vi "WholeImageROIFitBackUp.vi"(3 "Select directory with EYE files":path=path "E:/junk/EYEFiles") -> ()   [LabVIEW 2022 SP3]
uses:
  <vilib>/Utility/file.llb/Read From Spreadsheet File (DBL).vi
  <vilib>/Utility/file.llb/Write To Spreadsheet File (DBL).vi
  <vilib>/Analysis/NI_AALBase.lvlib
  <vilib>/Analysis/baseanly.llb/Mean (DBL).vi
panel:
  out "Sector as data array":dbl[][](graph)
  out "min value":dbl
  out "max value":dbl
  in  "ExitSendCmd":bool
  in  "Calculate TTIs":bool
  out "Current File":string
  out "Col scores":dbl[][](graph)
  out "Col midband":dbl[][](graph)
  out "NN Score":dbl[][](graph)
  in  "Tab Control":T1(tab)=enum."Image Prams"
  in  "Corrections":T2(ring)=enum."att correction"
  in  "type of cal file":u16(ring) items=["Normal Cal File", "Cross Cal File", "No cal file"]
  out "Cal File Att":string
  out "RF File Att":string
  in  "Cal File Name":string
  in  "Fit band":T3 {"center freq" format="%.2f"; "stop freq" format="%.2f"; "start" format="%.2f"}
  in  "Use Info In Header?":bool=TRUE
  in  "Lines to Avg":i32=1
  in  "Pts between window":i32=8
  in  "Pts in window":i32=64
  in  "sound speed":dbl=1.5 format="%.2f"
  in  "Padded FFT size":u16(ring)=6 items=["next 2^n", "8", "16", "32", "64", "128", "256", "512"]
  in  "Att (db/ cm MHz)":dbl=0.5 format="%.2f"
  in  "Add Switch Noise?":bool
  in  "Log scaling?":bool=TRUE
  out "Fit array":T4
  in  "Sub-Band Filter":T5={"Fit band"={"low freq"=3.5, "high freq"=8.0, "center freq"=5.75}, "MB threshold"=0.0, "Sub-Band Filter?"=FALSE} {"MB threshold" format="%.2f"; "Fit band"."center freq" format="%.2f"; "Fit band"."high freq" format="%.2f"; "Fit band"."low freq" format="%.2f"}
  in  "CQPrams":T6={"Data System params"={"sample freq (MHz)"=50.0, "focal length (mm)"=32.0, "aperature radius (mm)"=3.5, "pts in window"=64.0}, "Show CQ^2 image?"=FALSE, "Save?"=FALSE} {"Data System params"."pts in window" format="%.2f"; "Data System params"."aperature radius (mm)" format="%.2f"; "Data System params"."focal length (mm)" format="%.2f"; "Data System params"."sample freq (MHz)" format="%.2f"}
  out "CQ^2":ext[][](graph)
  out "radius (micron)":sgl[][](graph)
  in  "Range Params":T7={"mb max"=-20.0, "mb min"=-70.0, "slope max"=8.0, "slope min"=-8.0, "int max"=5.0, "int min"=-85.0} {"int min" format="%.2f"; "int max" format="%.2f"; "slope min" format="%.2f"; "slope max" format="%.2f"; "mb min" format="%.2f"; "mb max" format="%.2f"}
  in  "Final Sector Image Size":T8={"x"=346, "y"=240, "Trim image sides?"=FALSE, "start trim"=45, "end trim line"=256}
  in  "Simple BMP":bool
  in  "Raw Data Formats":T9(ring)
  in  "Save Raw Results?":bool
  in  "PSA Value":dbl=8.7 format="%.2f"
  in  "Look Up Table":path=path "E:/junk/EYEFiles/99lktbl10-31.txt"
  in  "Create Score Image?":bool
  in  "thresholds":T10={"T1"=0.37, "T2"=0.38, "T3"=0.39, "T4"=0.4, "T5"=0.43} {"T5" scale=3.0..47.0; "T4" scale=3.0..47.0; "T3" scale=3.0..47.0; "T2" scale=3.0..47.0; "T1" scale=3.0..47.0}
  in  "Save Score Dat?":bool
  in  "Color Table":u32[](array[colorbox])=[0, 0, 65793, 131586, 197379, 263172, 328965, 394758, 460551, 526344, 592137, 657930, 723723, 789516, 855309, 921102, 986895, 1052688, 1118481, 1184274, 1250067, 1315860, 1381653, 1447446, 1513239, 1579032, 1644825, 1710618, 1776411, 1842204, 1907997, 1973790, 2039583, 2105376, 2171169, 2236962, 2302755, 2368548, 2434341, 2500134, 2565927, 2631720, 2697513, 2763306, 2829099, 2894892, 2960685, 3026478, 3092271, 3158064, 3223857, 3289650, 3355443, 3421236, 3487029, 3552822, 3618615, 3684408, 3750201, 3815994, 3881787, 3947580, 4013373, 4079166, 4144959, 4210752, 4276545, 4342338, 4408131, 4473924, 4539717, 4605510, 4671303, 4737096, 4802889, 4868682, 4934475, 5000268, 5066061, 5131854, 5197647, 5263440, 5329233, 5395026, 5460819, 5526612, 5592405, 5658198, 5723991, 5789784, 5855577, 5921370, 5987163, 6052956, 6118749, 6184542, 6250335, 6316128, 6381921, 6447714, 6513507, 6579300, 6645093, 6710886, 6776679, 6842472, 6908265, 6974058, 7039851, 7105644, 7171437, 7237230, 7303023, 7368816, 7434609, 7500402, 7566195, 7631988, 7697781, 7763574, 7829367, 7895160, 7960953, 8026746, 8092539, 8158332, 8224125, 8289918, 8355711, 8421504, 8487297, 8553090, 8618883, 8684676, 8750469, 8816262, 8882055, 8947848, 9013641, 9079434, 9145227, 9211020, 9276813, 9342606, 9408399, 9474192, 9539985, 9605778, 9671571, 9737364, 9803157, 9868950, 9934743, 10000536, 10066329, 10132122, 10197915, 10263708, 10329501, 10395294, 10461087, 10526880, 10592673, 10658466, 10724259, 10790052, 10855845, 10921638, 10987431, 11053224, 11119017, 11184810, 11250603, 11316396, 11382189, 11447982, 11513775, 11579568, 11645361, 11711154, 11776947, 11842740, 11908533, 11974326, 12040119, 12105912, 12171705, 12237498, 12303291, 12369084, 12434877, 12500670, 12566463, 12632256, 12698049, 12763842, 12829635, 12895428, 12961221, 13027014, 13092807, 13158600, 13224393, 13290186, 13355979, 13421772, 13487565, 13553358, 13619151, 13684944, 13750737, 13816530, 13882323, 13948116, 14013909, 14079702, 14145495, 14211288, 14277081, 14342874, 14408667, 14474460, 14540253, 14606046, 14671839, 14737632, 14803425, 14869218, 14935011, 15000804, 15066597, 15132390, 15198183, 15263976, 15329769, 15395562, 15461355, 15527148, 15592941, 15658734, 15724527, 15790320, 15856113, 15921906, 15987699, 16053492, 16119285, 16185078, 16250871, 16316664, 16382457, 6352640, 12058434, 16770066, 16758546, 16711731]
  in  "Data Set":i32
  in  "Rescale Thresh":bool
  in  "Create Cross Cal?":bool
  out "Cross Cal":dbl[][](graph)
  in  "Ring":u16(ring) items=["Select Files in Listbox", "Choose list of files"]
  in  "File Names":i32[](listbox)
  out "raw data":i16[][](graph)
  out "midband fit":dbl[][](graph)
  out "intercept":dbl[][](graph)
  out "slope":dbl[][](graph)
  # "© 2000-2010 Riverside Research Institute"
  # "Parameters to select before hitting \"Calculate TTIs\"."
  # "Spectrum Fit Parameters"
  # "Select to add back in switch noise from B&K Hawk machine."
  # "Values used to make image."
  # "Optional suband filter which is really never used and may not function properly in current version."
  # "Can be selected after calculating TTIs"
  # "CQPrams files are saved as spreadsheet files. Radius file is in microns and cq^2 file is in dB."
  # "Save raw data and MB side by side"
  # "Score images need to be created with all corrections applied data. This means a cross cal file with attenutation corrections for Hawk and Hitachi, and data base corrections for B&K 3535.\n\nFinal image size settings are in Image Prams tab. Data saves as a BMP file in sector format.\n\nCreate Score Image? will color code images and Save Score Dat? will save images as BMPs."
  # "If making Cross Cal file, select No cal file option and att correction."
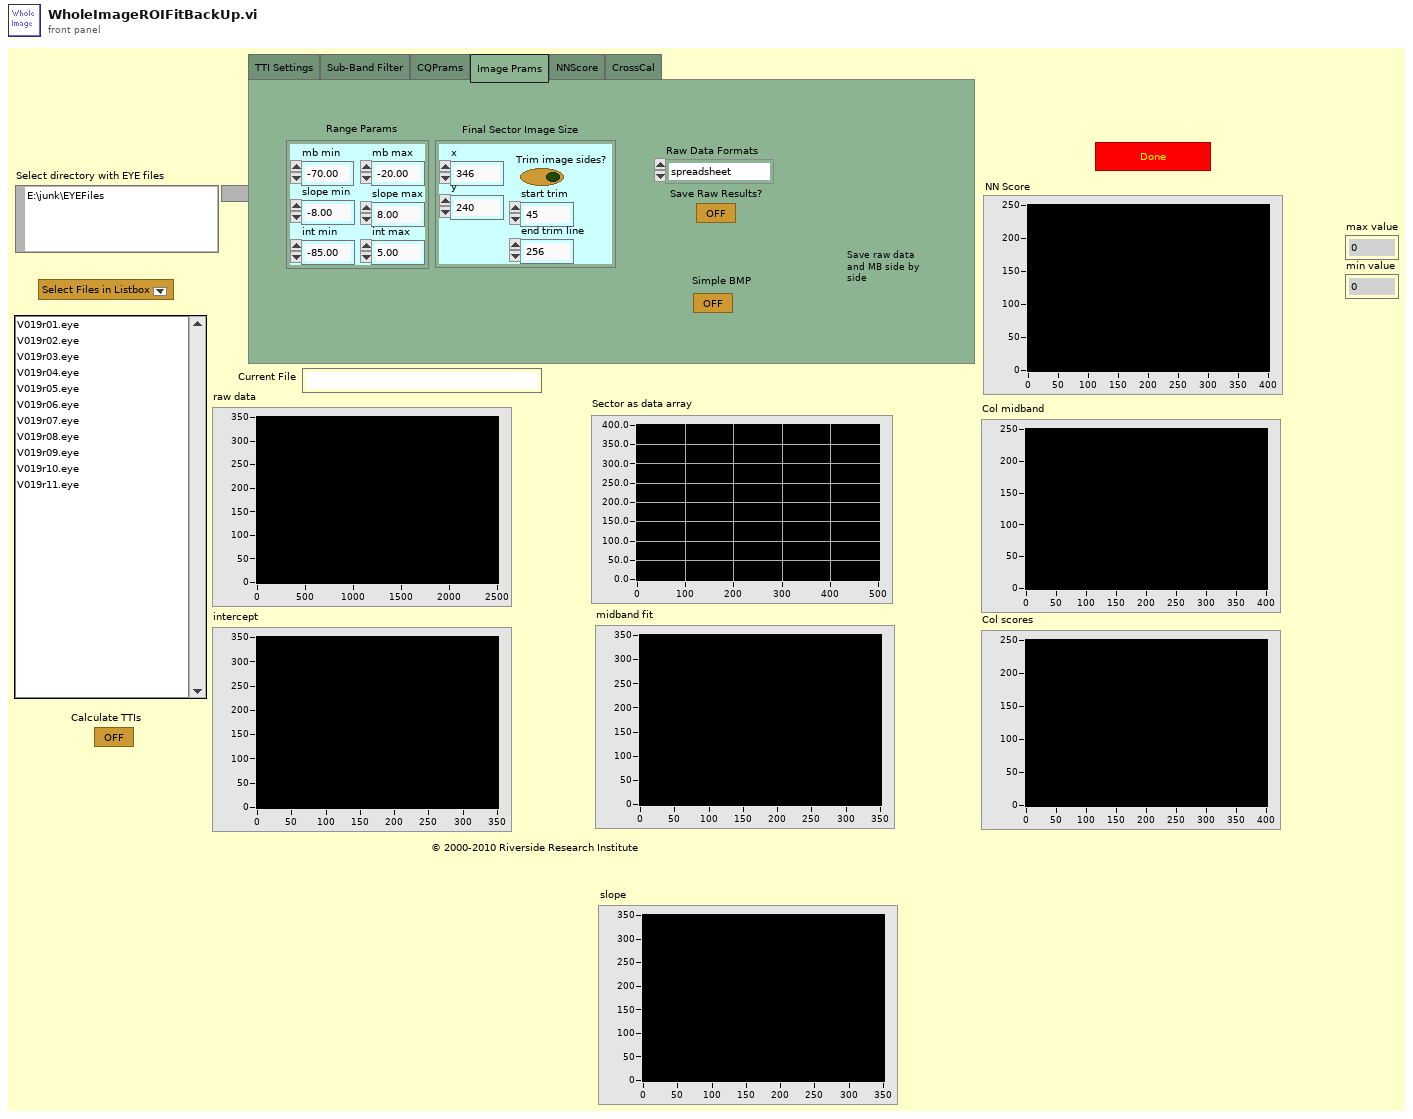
[diagram p1: front panel]
types:
  T1 = enum32{"TTI Settings", "Sub-Band Filter", "CQPrams", "Image Prams", "NNScore", "CrossCal"}
  T2 = enum16{"no att correction", "att correction", "B&K 3535, TGC & att corr"}
  T3 = cluster{"start":dbl, "stop freq":dbl, "center freq":dbl}
  T4 = cluster{"x length":i32, "y length":i32, "ROIs in x":i32, "ROIs in y":i32}
  T5 = cluster{"Fit band":cluster{"low freq":dbl, "high freq":dbl, "center freq":dbl}, "MB threshold":dbl, "Sub-Band Filter?":bool}
  T6 = cluster{"Data System params":cluster{"sample freq (MHz)":dbl, "focal length (mm)":sgl, "aperature radius (mm)":sgl, "pts in window":dbl}, "Show CQ^2 image?":bool, "Save?":bool}
  T7 = cluster{"mb max":dbl, "mb min":dbl, "slope max":dbl, "slope min":dbl, "int max":dbl, "int min":dbl}
  T8 = cluster{"x":i32, "y":i32, "Trim image sides?":bool, "start trim":i32, "end trim line":i32}
  T9 = enum16{"spreadsheet", "8 bit byte file", "sector byte file", "8 bit BMP file", "sector 8 bit BMP file"}
  T10 = cluster{"T1":dbl, "T2":dbl, "T3":dbl, "T4":dbl, "T5":dbl}
  T11 = cluster{"# rf points per line":u16, "# lines per scan":u16, "sample rate MHz":u16, "# A/D bits":u16, "# bytes per A/D":u16, "TGC Flag":u16, "A/D Type":string}
  T12 = cluster{"bandwidth":sgl, "center freq":sgl, "start freq":sgl, "ID":i32}
  T13 = cluster{"delay":sgl, "pivot distance":sgl, "sector scan angle":sgl, "operator":string, "Scan Mode":string, "location":string}
  T14 = cluster{"RF file name":string, "RF file att":string, "RF cal file name":string, "RF cal file att":string}
  T15 = cluster{"RF cal file name":string, "RF file att":string, "Cal File Name":string, "RF cal file att":string}
  T16 = cluster{"start freq":sgl, sgl, "center freq":sgl}
  T17 = cluster{"Pts in window":i32, "Lines to Avg":i32, dbl, "# lines per scan":u16}
  T18 = cluster{"slope (m)":dbl[][], "intercept (b)":dbl[][], "midband fit":dbl[][], "pts in fit":dbl}
  T19 = cluster{"slope (m)":dbl, "m stand dev":dbl, "intercept (b)":dbl, "b stand dev":dbl, "MSE":dbl, "midband fit":dbl, "pts in fit":dbl}
  T20 = typedef "imagedata.ctl" = cluster{"image type":i32, "image depth":i32, "image":u8[], "mask":u8[], "colors":u32[], "Rectangle":cluster{"left":i16, "top":i16, "right":i16, "bottom":i16}}
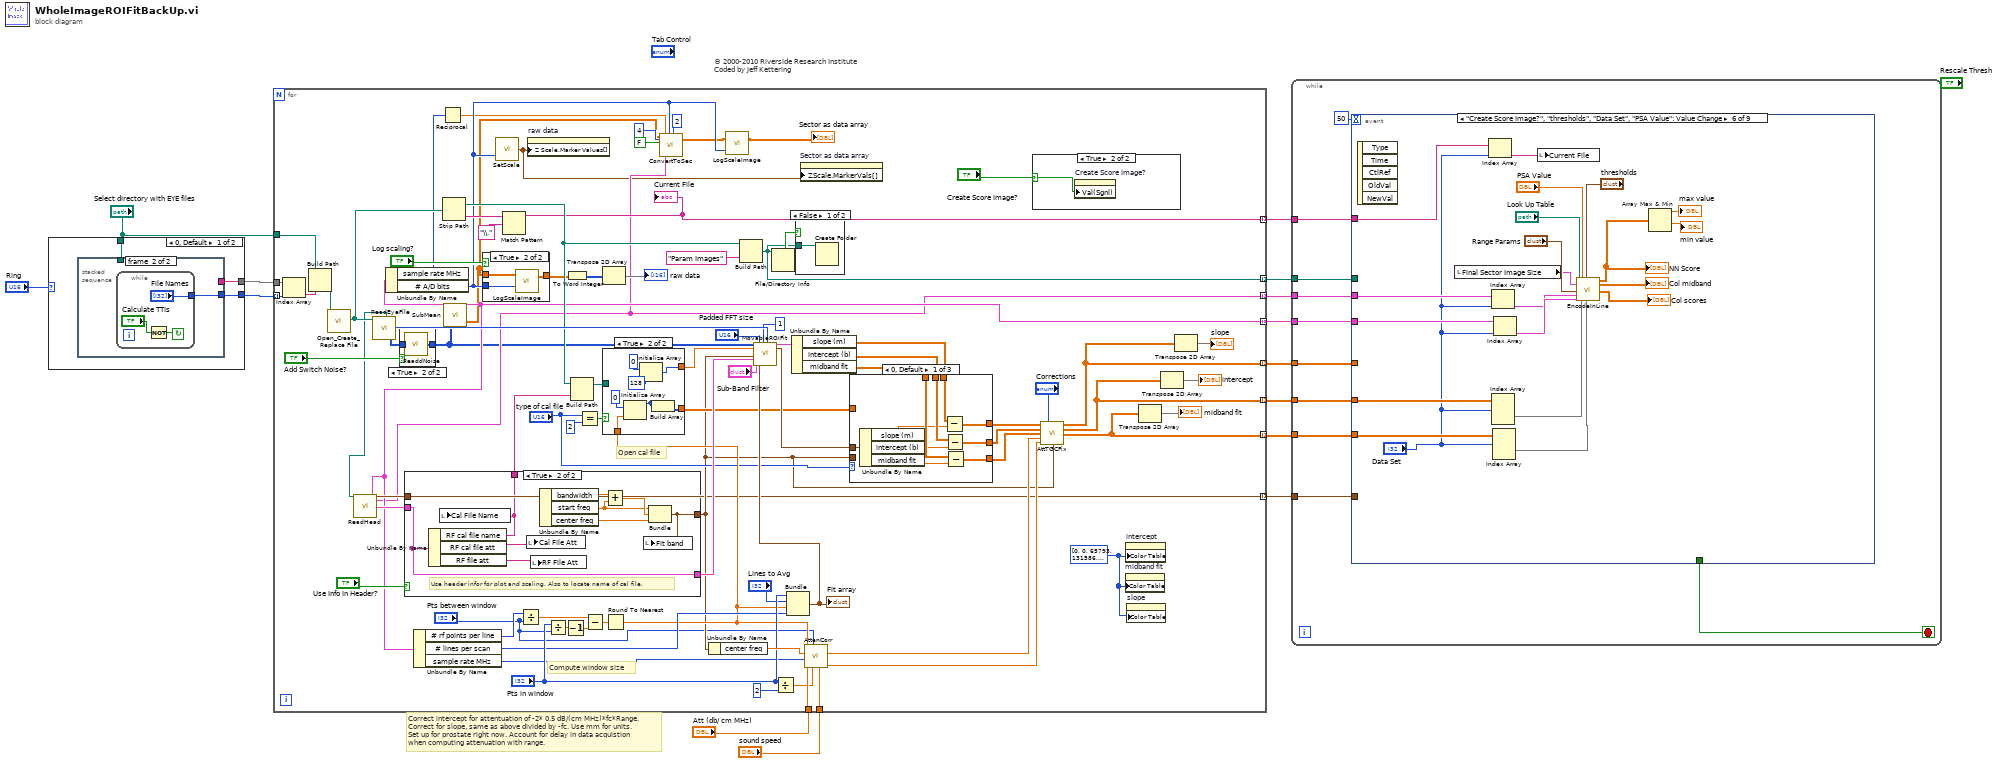
[diagram p0: block diagram]
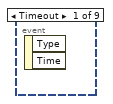
[diagram p2: hidden frame]
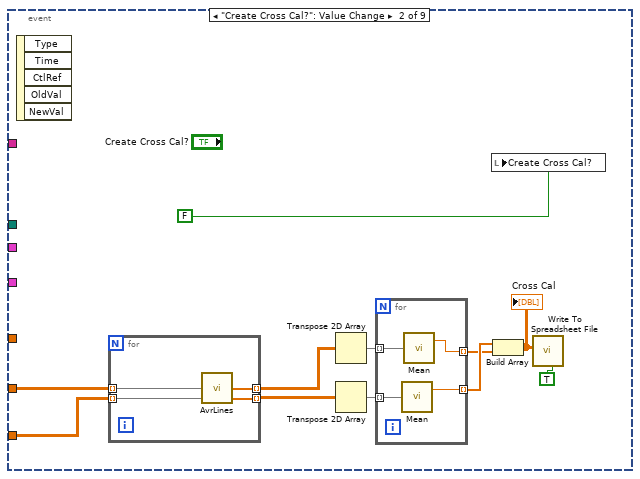
[diagram p3: hidden frame]
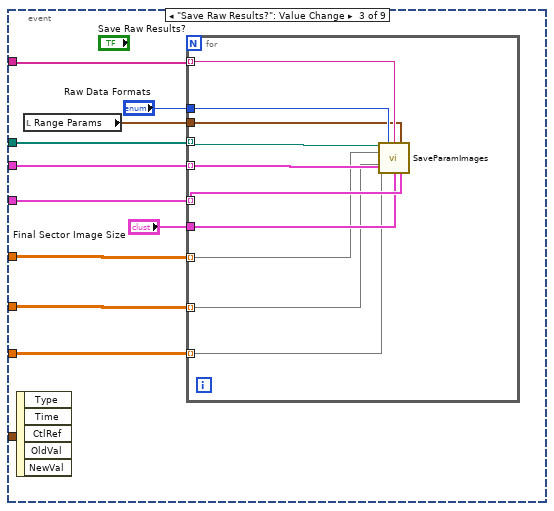
[diagram p4: hidden frame]
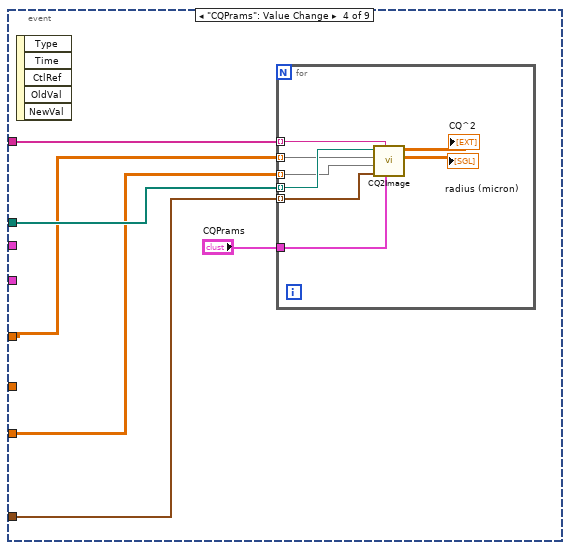
[diagram p5: hidden frame]
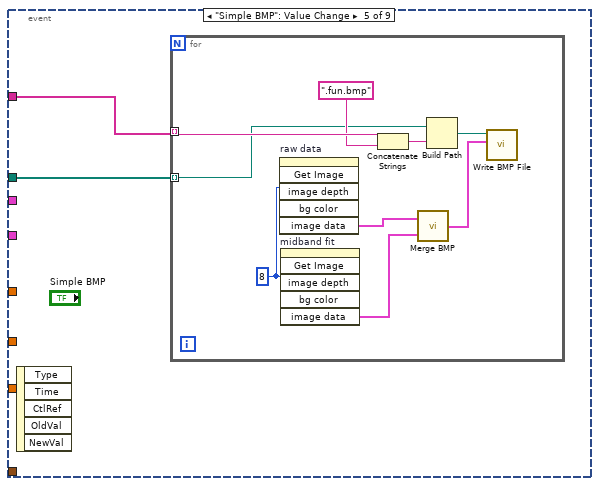
[diagram p6: hidden frame]
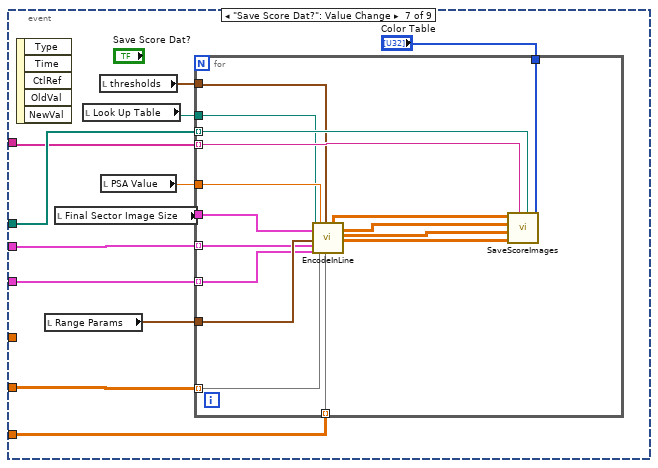
[diagram p7: hidden frame]
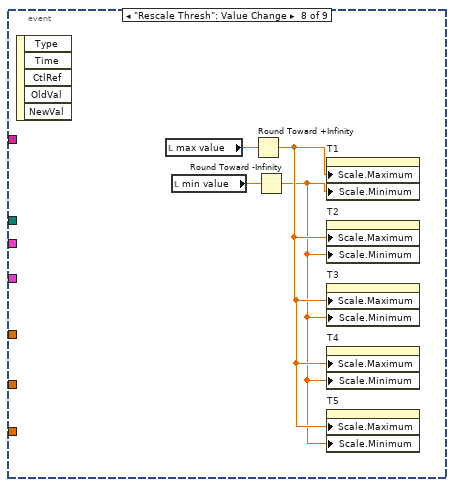
[diagram p8: hidden frame]
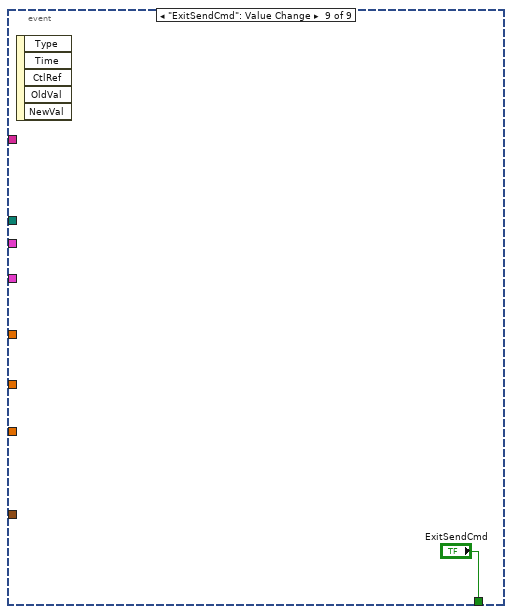
[diagram p9: hidden frame]
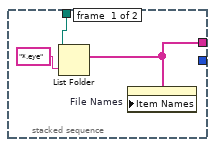
[diagram p10: hidden frame]
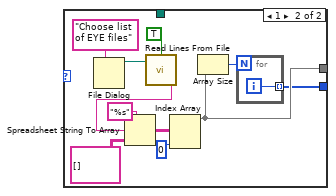
[diagram p11: hidden frame]
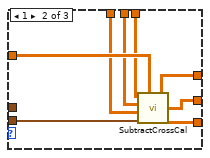
[diagram p15: hidden frame]
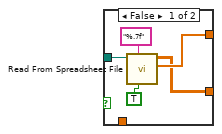
[diagram p17: hidden frame]
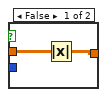
[diagram p18: hidden frame]
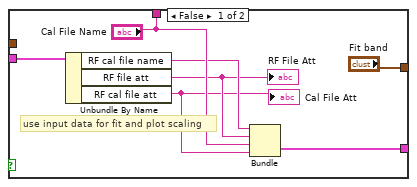
[diagram p19: hidden frame]
diagram:
  # "© 2000-2010 Riverside Research Institute\nCoded by Jeff Kettering"
  # "Correct intercept for attentuation of -2* 0.5 dB/(cm MHz)*fc*Range.\nCorrect for slope, same as above divided by -fc. Use mm for units. \nSet up for prostate right now. Account for delay in data acquistion when computing attenuation with range."
  n1 = case shown="0, Default" "Ring" {
    tunnel: [w17 w27] -> w14
    tunnel: "Select directory with EYE files" -> [w16 _]
    tunnel: [w15 w25] -> w13
    frame 0, Default {
      n2 = stacked-sequence {
        tunnel: [w19 _] -> w17
        tunnel: w16 -> [w18 _]
        tunnel: [_ w21] -> w15
        frame #0 {
          n3 = List Folder(path=w18, pattern="*.eye") -> (filenames=w19:string[])  [unwired: 1 in, 4 out]
          n4 = property on="File Names" class="LstBox (strict)"("Item Names"=w19) -> ()  [unwired: 2 in, 2 out]
        }
        frame #1 {
          n5 = while {
            tunnel: ["File Names"] -> w21
            stop <- w22 continue-if-true
            n6 = Not(x="Calculate TTIs") -> (.not. x?=w22:bool)
          }
        }
      }
    }
    frame 1 {
      n7 = File Dialog(7:"Choose list of EYE files" ("prompt")) -> (3:w33:path)  [unwired: 1 in, 8 out]
      n8 = call <vilib>:"Read Lines From File.vi"("convert eol? (no:F)"=TRUE, "file path (dialog if empty)"=w33) -> ("line string"=w28:string)  [unwired: 1 in, 6 out]
      n9 = Spreadsheet String To Array(format string="%s", spreadsheet string=w28, array type (2D Dbl)=string[][] [] ("Array Constant")) -> (array=w32:string[][])  [unwired: 1 in]
      n10 = Index Array(array=w32, index (col)=0) -> (element=w27:string[])  [unwired: 1 in]
      n11 = Array Size(array=w27) -> (size(s)=w26:i32)
      n12 = for {
        N: w26 -> [_]
        tunnel: [w36] -> w25 mode=indexing
        i -> [w36]
      }
    }
  }
  n13 = for {
    tunnel: w14 -> [w111]
    tunnel: "Select directory with EYE files" -> [w110]
    tunnel: w13 -> [w106] mode=indexing
    tunnel: "Att (db/ cm MHz)" -> [w96]
    tunnel: "sound speed" -> [w68]
    tunnel: [w61] -> w8 mode=indexing
    tunnel: [w60] -> w7 mode=indexing
    tunnel: [w55] -> w6 mode=indexing
    tunnel: [w56] -> w5 mode=indexing
    tunnel: [w57] -> w4 mode=indexing
    tunnel: [w54] -> w3 mode=indexing
    tunnel: [w46] -> w2 mode=indexing
    tunnel: [w53] -> w1 mode=indexing
    w67 = u32[] [0, 0, 65793, 131586, 197379, 263172, 328965, 394758, 460551, 526344, 592137, 657930, 723723, 789516, 855309, 921102, 986895, 1052688, 1118481, 1184274, 1250067, 1315860, 1381653, 1447446, 1513239, 1579032, 1644825, 1710618, 1776411, 1842204, 1907997, 1973790, 2039583, 2105376, 2171169, 2236962, 2302755, 2368548, 2434341, 2500134, 2565927, 2631720, 2697513, 2763306, 2829099, 2894892, 2960685, 3026478, 3092271, 3158064, 3223857, 3289650, 3355443, 3421236, 3487029, 3552822, 3618615, 3684408, 3750201, 3815994, 3881787, 3947580, 4013373, 4079166, 4144959, 4210752, 4276545, 4342338, 4408131, 4473924, 4539717, 4605510, 4671303, 4737096, 4802889, 4868682, 4934475, 5000268, 5066061, 5131854, 5197647, 5263440, 5329233, 5395026, 5460819, 5526612, 5592405, 5658198, 5723991, 5789784, 5855577, 5921370, 5987163, 6052956, 6118749, 6184542, 6250335, 6316128, 6381921, 6447714, 6513507, 6579300, 6645093, 6710886, 6776679, 6842472, 6908265, 6974058, 7039851, 7105644, 7171437, 7237230, 7303023, 7368816, 7434609, 7500402, 7566195, 7631988, 7697781, 7763574, 7829367, 7895160, 7960953, 8026746, 8092539, 8158332, 8224125, 8289918, 8355711, 8421504, 8487297, 8553090, 8618883, 8684676, 8750469, 8816262, 8882055, 8947848, 9013641, 9079434, 9145227, 9211020, 9276813, 9342606, 9408399, 9474192, 9539985, 9605778, 9671571, 9737364, 9803157, 9868950, 9934743, 10000536, 10066329, 10132122, 10197915, 10263708, 10329501, 10395294, 10461087, 10526880, 10592673, 10658466, 10724259, 10790052, 10855845, 10921638, 10987431, 11053224, 11119017, 11184810, 11250603, 11316396, 11382189, 11447982, 11513775, 11579568, 11645361, 11711154, 11776947, 11842740, 11908533, 11974326, 12040119, 12105912, 12171705, 12237498, 12303291, 12369084, 12434877, 12500670, 12566463, 12632256, 12698049, 12763842, 12829635, 12895428, 12961221, 13027014, 13092807, 13158600, 13224393, 13290186, 13355979, 13421772, 13487565, 13553358, 13619151, 13684944, 13750737, 13816530, 13882323, 13948116, 14013909, 14079702, 14145495, 14211288, 14277081, 14342874, 14408667, 14474460, 14540253, 14606046, 14671839, 14737632, 14803425, 14869218, 14935011, 15000804, 15066597, 15132390, 15198183, 15263976, 15329769, 15395562, 15461355, 15527148, 15592941, 15658734, 15724527, 15790320, 15856113, 15921906, 15987699, 16053492, 16119285, 16185078, 16250871, 16316664, 16382457, 16448250, 16514043, 16579836, 16645629, 16711680] ("Color Table")
    # "Compute window size"
    # "Open cal file"
    n14 = Index Array(array=w111, index=w106) -> (element=w109:string)
    n15 = Build Path(base path=w110, name or relative path=w109) -> (appended path=w108:path)
    n16 = call <vilib>:"Open_Create_Replace File.vi"("file path"=w108) -> ("new file path"=w107:path)  [unwired: 5 in, 5 out]
    n17 = call "ReadEyeFile.vi"("new file path"=w107) -> ("new path out"=w66:path, "2-D data array"=w75:i16[][], "sample rate MHz"=w114:u16)  [unwired: 1 in, 15 out]
    n18 = call "ReadHead.vi"("new file path"=w66) -> ("A/D info"=w53:T11, "Tranducer Info"=w57:T12, "Scan Info"=w46:T13, "RF Info"=w120:T14)  [unwired: 15 out]
    n19 = Unbundle By Name(w53) -> ("sample rate MHz"=w45:u16, "# A/D bits"=w43:u16)
    n20 = case shown="True" "Add Switch Noise?" {
      tunnel: [w123 w125] -> w37
      tunnel: w75 -> [w123 w124]
      frame False {
      }
      frame True {
        n21 = call "ReaddNoise.vi"("Data in"=w124) -> ("Data out"=w125:i16[][])
      }
    }
    n22 = case shown="True" "Use Info In Header?" {
      tunnel: w57 -> [_ w181]
      tunnel: ["Fit band" w178] -> w69
      tunnel: w120 -> [w169 w172]
      tunnel: ["Cal File Name" w173] -> w117
      tunnel: [w167 w172] -> w112
      frame False {
        # "use input data for fit and plot scaling"
        n23 = Unbundle By Name(w169) -> ("RF cal file name"=w168:string, "RF file att"=w166:string, "RF cal file att"=w165:string)
        "RF File Att" <- w166
        "Cal File Att" <- w165
        n24 = Bundle("RF cal file name"=w168, "RF file att"=w166, "Cal File Name"="Cal File Name", "RF cal file att"=w165) -> (w167:T15)  [unwired: 1 out]
      }
      frame True {
        # "Use header infor for plot and scaling. Also to locate name of cal file."
        n25 = Unbundle By Name(w172) -> ("RF cal file name"=w173:string, "RF cal file att"=w175:string, "RF file att"=w174:string)
        n26 = local write "Cal File Name"(w173) -> ()
        n27 = local write "Cal File Att"(w175) -> ()
        n28 = local write "RF File Att"(w174) -> ()
        n29 = Unbundle By Name(w181) -> ("bandwidth"=w180:sgl, "start freq"=w176:sgl, "center freq"=w179:sgl)
        n30 = Add(x=w180, y=w176) -> (x+y=w177:sgl)
        n31 = Bundle("start freq"=w176, w177, "center freq"=w179) -> (w178:T16)  [unwired: 1 out]
        n32 = local write "Fit band"(w178) -> ()
      }
    }
    n33 = Unbundle By Name(w53) -> ("# rf points per line"=w98:u16, "# lines per scan"=w73:u16, "sample rate MHz"=w89:u16)
    n34 = Reciprocal(x=w45) -> (1/x=w42:dbl)
    n35 = Strip Path(path=w107) -> (stripped path=w85:path, name=w82:string)
    n36 = call "SubMean.vi"("Scan Data In"=w37) -> ("Array"=w38:dbl[][])  [unwired: 1 in, 1 out]
    n37 = case shown="True" "Log scaling?" {
      tunnel: [w161 w164] -> w47
      tunnel: w38 -> [w160 w163]
      tunnel: w43 -> [_ w162]
      frame False {
        n38 = Absolute Value(x=w160) -> (abs(x)=w161:dbl[][])
      }
      frame True {
        n39 = call "LogScaleImage.vi"("A/D bits"=w162, "input array"=w163) -> ("log scale image"=w164:dbl[][])  [unwired: 1 out]
      }
    }
    n40 = call "SetScale.vi"("# A/D bits"=w43) -> ("Array"=w39:cluster{dbl, u32}[])  [unwired: 1 in]
    n41 = Match Pattern(string=w82, regular expression="\\." ("search char (-)")) -> (before substring=w61:string)  [unwired: 4 out]
    "Current File" <- w61
    n42 = Divide(x=w98, y="Pts between window") -> (x/y=w100:dbl)
    n43 = property on="raw data" class="IntGraph (strict)"("Z Scale.Marker Values[]"=w39) -> ()  [unwired: 2 in, 2 out]
    n44 = Divide(x="Pts in window", y="Pts between window") -> (x/y=w91:dbl)
    n45 = Decrement(x=w91) -> (x-1=w90:dbl)
    n46 = To Word Integer(number=w47) -> (16bit integer=w64:i16[][])
    n47 = Build Path(base path=w85, name or relative path=w117) -> (appended path=w105:path)
    n48 = Equal?(x="type of cal file", y=2) -> (x = y?=w97:bool)
    n49 = Subtract(x=w100, y=w90) -> (x-y=w99:dbl)
    n50 = Transpose 2D Array(2D array=w64) -> (transposed array=→"raw data":i16[][])
    n51 = Round To Nearest(number=w99) -> (nearest integer value=w72:dbl)
    n52 = case shown="True" w97 {
      tunnel: w105 -> [w152 _]
      tunnel: [w149 w157] -> w119
      tunnel: [w148 w153] -> w70
      tunnel: w72 -> [_ w156]
      frame False {
        n53 = call-poly <vilib>:"Read From Spreadsheet File.vi"("transpose (no:F)"=TRUE, "format (%.3f)"="%.7f", "file path (dialog if empty)"=w152) -> ("first row"=w149:dbl[], "all rows"=w148:dbl[][])  [unwired: 1 in, 6 out]
      }
      frame True {
        n54 = Initialize Array(0, w156) -> (w154:i32[])
        n55 = Initialize Array(0, 128) -> (w157:i32[])
        n56 = Build Array(w154, w154) -> (w153:i32[][])
      }
    }
    n57 = call "ConvertToSec.vi"("raw image data in"=w38, "reduce pts by factor of"=4, "Add Lines"=FALSE ("no oversample?"), "Time between rf pts\nmicros"=w42, "Scan Info"=w46, "Abs?"=w43, "Smooth factor"=2) -> ("raw sector out"=w41:dbl[][])  [unwired: 4 in, 8 out]
    n58 = Unbundle By Name(w69) -> ("center freq"=w95:dbl)
    n59 = call "LogScaleImage.vi"("A/D bits"=w43, "input array"=w41) -> ("log scale image"=→"Sector as data array":dbl[][])  [unwired: 1 out]
    n60 = Build Path(base path=w85, name or relative path="Param Images") -> (appended path=w60:path)
    n61 = File/Directory Info(path=w60) -> (directory=w86:bool)  [unwired: 1 in, 6 out]
    n62 = Divide(x="Pts in window", y=2) -> (x/y=w94:dbl)
    n63 = Bundle("Pts in window"="Pts in window", "Lines to Avg"="Lines to Avg", w72, "# lines per scan"=w73) -> (w76:T17)  [unwired: 1 out]
    "Fit array" <- w76
    n64 = call "MovableROIFit.vi"("input array"=w37, "calibration data"=w119, "Fit band"=w69, "RF Info"=w112, "Sub-Band Filter"="Sub-Band Filter", "FFT size for"="Padded FFT size", "Fit array"=w76, "Proc Method"=1, "freq (MHz)"=w114) -> ("Raw Fit Data"=w116:T18, "Cal params"=w115:T19)  [unwired: 4 in, 5 out]
    n65 = Unbundle By Name(w116) -> ("slope (m)"=w101:dbl[][], "intercept (b)"=w102:dbl[][], "midband fit"=w103:dbl[][])
    n66 = case shown="False" w86 {
      tunnel: w60 -> [w126 _]
      frame False {
        n67 = Create Folder(path (use dialog)=w126) -> ()  [unwired: 1 in, 4 out]
      }
      frame True {
      }
    }
    n68 = property on="Sector as data array" class="IntGraph (strict)"("ZScale.MarkerVals[]"=w39) -> ()  [unwired: 2 in, 2 out]
    n69 = call "AttenCorr.vi"("sound speed"=w68, "Offset"=w94, "Step size"="Pts between window", "Attenuation (db/ cm MHz)"=w96, "Sampling Freq (MHz)"=w89, "Center Freq"=w95, "ROIs in x"=w72) -> ("slope correction"=w77:dbl[], "midband correction"=w78:dbl[])  [unwired: 2 out]
    n70 = case shown="0, Default" "type of cal file" {
      tunnel: w115 -> [w136 _ _]
      tunnel: w103 -> [w135 w139 w146]
      tunnel: [w134 w143 w146] -> w79
      tunnel: w102 -> [w133 w138 w147]
      tunnel: [w132 w142 w147] -> w80
      tunnel: w101 -> [w131 w137 w145]
      tunnel: [w130 w141 w145] -> w81
      tunnel: w69 -> [_ w144 _]
      tunnel: w70 -> [_ w140 _]
      frame 0, Default {
        n71 = Unbundle By Name(w136) -> ("slope (m)"=w129:dbl, "intercept (b)"=w128:dbl, "midband fit"=w127:dbl)
        n72 = Subtract(x=w131, y=w129) -> (x-y=w130:dbl[][])
        n73 = Subtract(x=w133, y=w128) -> (x-y=w132:dbl[][])
        n74 = Subtract(x=w135, y=w127) -> (x-y=w134:dbl[][])
      }
      frame 1 {
        n75 = call "SubtractCrossCal.vi"("slope (m)"=w137, "intercept (b) out"=w138, "midband fit in"=w139, "Fit band"=w144, "Cross Cal"=w140) -> ("slope out"=w141:dbl[][], "intercept out"=w142:dbl[][], "midband fitout"=w143:dbl[][])
      }
      frame 2 {
      }
    }
    n76 = case shown="True" "Create Score Image?" {
      selector: "Create Score Image?" -> [_ w122]
      frame False {
      }
      frame True {
        n77 = property on="Create Score Image?" class="Bool (strict)"("Val(Sgnl)"=w122) -> ()  [unwired: 2 in, 2 out]
      }
    }
    n78 = call "AttTGCFix.vi"("slope (m)"=w81, "Corrections"="Corrections", "intercept (b) out"=w80, "midband fit in"=w79, "midband correction"=w78, "slope correction"=w77, "Fit band"=w69) -> ("slope"=w55:dbl[][], "intercept"=w54:dbl[][], "midband fit"=w56:dbl[][])  [unwired: 1 in, 5 out]
    n79 = property on="midband fit" class="IntGraph (strict)"("Color Table"=w67) -> ()  [unwired: 2 in, 2 out]
    n80 = property on="intercept" class="IntGraph (strict)"("Color Table"=w67) -> ()  [unwired: 2 in, 2 out]
    n81 = property on="slope" class="IntGraph (strict)"("Color Table"=w67) -> ()  [unwired: 2 in, 2 out]
    n82 = Transpose 2D Array(2D array=w56) -> (transposed array=→"midband fit":dbl[][])
    n83 = Transpose 2D Array(2D array=w54) -> (transposed array=→"intercept":dbl[][])
    n84 = Transpose 2D Array(2D array=w55) -> (transposed array=→"slope":dbl[][])
  }
  n85 = while {
    tunnel: w8 -> [w191]
    tunnel: w7 -> [w190]
    tunnel: w6 -> [w189]
    tunnel: w5 -> [w188]
    tunnel: w4 -> [w187]
    tunnel: w3 -> [w186]
    tunnel: w2 -> [w185]
    tunnel: w1 -> [w184]
    stop <- w182 stop-if-true
    n86 = event shown="[5] \"Create Score Image?\", \"thresholds\", \"Data Set\", \"PSA Value\": Value Change" {
      selector: _ -> [_ _ _ _ _ _ _ _ _]
      dyn-events: _ -> [_ _ _ _ _ _ _ _ _]
      timeout: 50 -> [_ _ _ _ _ _ _ _ _]
      tunnel: w191 -> [_ _ w220 w231 w245 w261 w287 _ _]
      tunnel: w190 -> [_ _ w218 w235 w246 _ w288 _ _]
      tunnel: w189 -> [_ _ w215 w234 _ _ _ _ _]
      tunnel: w188 -> [_ w193 w213 w233 _ w267 w283 _ _]
      tunnel: w187 -> [_ _ _ w232 _ _ _ _ _]
      tunnel: w186 -> [_ w194 w214 _ _ w269 w284 _ _]
      tunnel: w185 -> [_ _ w217 _ _ w263 w286 _ _]
      tunnel: w184 -> [_ _ w216 _ _ w265 w285 _ _]
      tunnel: [_ _ _ _ _ _ _ _ "ExitSendCmd"] -> w182
      event Timeout {
        n87 = event-data() -> ()  [unwired: 1 in, 2 out]
      }
      event "Create Cross Cal?": Value Change {
        n88 = event-data() -> ()  [unwired: 1 in, 5 out]
        n89 = for {
          tunnel: w194 -> [w210] mode=indexing
          tunnel: w193 -> [w209] mode=indexing
          tunnel: [w208] -> w196 mode=indexing
          tunnel: [w207] -> w195 mode=indexing
          n90 = call "AvrLines.vi"("midband fit in"=w209, "intercept (b) in"=w210) -> ("midband avr"=w207:dbl[], "intercept avr"=w208:dbl[])  [unwired: 1 in, 1 out]
        }
        n91 = Transpose 2D Array(2D array=w196) -> (transposed array=w202:dbl[][])
        n92 = Transpose 2D Array(2D array=w195) -> (transposed array=w201:dbl[][])
        n93 = for {
          tunnel: w201 -> [w206] mode=indexing
          tunnel: w202 -> [w205] mode=indexing
          tunnel: [w204] -> w198 mode=indexing
          tunnel: [w203] -> w199 mode=indexing
          n94 = call-poly <vilib>:"Mean.vi"("X"=w206) -> ("mean"=w203:dbl)  [unwired: 1 out]
          n95 = call-poly <vilib>:"Mean.vi"("X"=w205) -> ("mean"=w204:dbl)  [unwired: 1 out]
        }
        n96 = local write "Create Cross Cal?"(FALSE) -> ()
        n97 = Build Array(w199, w198) -> (w197:dbl[][])
        "Cross Cal" <- w197
        n98 = call-poly <vilib>:"Write To Spreadsheet File.vi"("transpose? (no:F)"=TRUE, "2D data"=w197) -> ()  [unwired: 4 in, 3 out]
      }
      event "Save Raw Results?": Value Change {
        n99 = event-data() -> ()  [unwired: 1 in, 5 out]
        n100 = local read "Range Params"() -> (w212:T7)
        n101 = for {
          tunnel: w220 -> [w230] mode=indexing
          tunnel: "Raw Data Formats" -> [w229]
          tunnel: w212 -> [w228]
          tunnel: w218 -> [w227] mode=indexing
          tunnel: w217 -> [w226] mode=indexing
          tunnel: w216 -> [w225] mode=indexing
          tunnel: "Final Sector Image Size" -> [w224]
          tunnel: w215 -> [w223] mode=indexing
          tunnel: w214 -> [w222] mode=indexing
          tunnel: w213 -> [w221] mode=indexing
          n102 = call "SaveParamImages.vi"("Directory Parh"=w227, "Data Formats"=w229, "file name"=w230, "Range Params"=w228, "slope"=w223, "intercept"=w222, "midband fit"=w221, 12:w226, "Final Image Size"=w224, 14:w225) -> ()  [unwired: 1 in, 5 out]
        }
      }
      event "CQPrams": Value Change {
        n103 = event-data() -> ()  [unwired: 1 in, 5 out]
        n104 = for {
          tunnel: "CQPrams" -> [w244]
          tunnel: w231 -> [w243] mode=indexing
          tunnel: w235 -> [w242] mode=indexing
          tunnel: w234 -> [w241] mode=indexing
          tunnel: w233 -> [w240] mode=indexing
          tunnel: w232 -> [w239] mode=indexing
          n105 = call "CQ2Image.vi"("CQPrams"=w244, "name"=w243, "Tranducer Info"=w239, "midband fit"=w240, "slope"=w241, "appended path"=w242) -> ("radius (micron)"=→"radius (micron)":sgl[][], "CQ^2"=→"CQ^2":ext[][])  [unwired: 2 out]
        }
      }
      event "Simple BMP": Value Change {
        n106 = event-data() -> ()  [unwired: 1 in, 5 out]
        n107 = for {
          tunnel: w245 -> [w255] mode=indexing
          tunnel: w246 -> [w247] mode=indexing
          w253 = 8
          n108 = invoke on="raw data" class="IntensityGraph (strict)" method="Get Image"("image depth"=w253) -> ("image data"=w250:T20)  [unwired: 5 in, 5 out]
          n109 = invoke on="midband fit" class="IntensityGraph (strict)" method="Get Image"("image depth"=w253) -> ("image data"=w249:T20)  [unwired: 5 in, 5 out]
          n110 = Concatenate Strings(w255, ".fun.bmp") -> (w251:string)
          n111 = call "Merge BMP.vi"("image two"=w249, "image one"=w250) -> ("Merged"=w248:T20)
          n112 = Build Path(base path=w247, name or relative path=w251) -> (appended path=w254:path)
          n113 = call <vilib>:"Write BMP File.vi"("image data"=w248, "path to BMP file"=w254) -> ()  [unwired: 1 in, 9 out]
        }
      }
      event "Create Score Image?", "thresholds", "Data Set", "PSA Value": Value Change {
        n114 = event-data() -> ()  [unwired: 1 in, 5 out]
        n115 = local read "Final Sector Image Size"() -> (w275:T8)
        n116 = Index Array(array=w261, index="Data Set") -> (element=w259:string)
        n117 = Index Array(array=w263, index="Data Set") -> (element=w262:T13)
        n118 = Index Array(array=w269, index (dim 0)="Data Set") -> (element=w268:dbl[][])  [unwired: 2 in]
        n119 = Index Array(array=w267, index (dim 0)="Data Set") -> (element=w266:dbl[][])  [unwired: 2 in]
        n120 = Index Array(array=w265, index="Data Set") -> (element=w264:T11)
        n121 = local write "Current File"(w259) -> ()
        n122 = call "EncodeInLine.vi"("Look Up Table"="Look Up Table", "Final Sector Image Size"=w275, "Range Params"="Range Params", "Header In"=w262, 5:w264, "PSA Value"="PSA Value", "intercept"=w268, "thresholds"="thresholds", "midband fit"=w266) -> ("Score Sector image"=w258:dbl[][], "Colored MB"=→"Col midband":dbl[][], "Colored Score"=→"Col scores":dbl[][])  [unwired: 1 in, 7 out]
        "NN Score" <- w258
        n123 = Array Max & Min(array=w258) -> (max value=→"max value":dbl, min value=→"min value":dbl)  [unwired: 2 out]
      }
      event "Save Score Dat?": Value Change {
        n124 = event-data() -> ()  [unwired: 1 in, 5 out]
        n125 = local read "Range Params"() -> (w278:T7)
        n126 = local read "Final Sector Image Size"() -> (w282:T8)
        n127 = local read "Look Up Table"() -> (w279:path)
        n128 = local read "thresholds"() -> (w280:T10)
        n129 = local read "PSA Value"() -> (w281:dbl)
        n130 = for {
          tunnel: w288 -> [w304] mode=indexing
          tunnel: w287 -> [w303] mode=indexing
          tunnel: w278 -> [w302]
          tunnel: w282 -> [w301]
          tunnel: w286 -> [w300] mode=indexing
          tunnel: w285 -> [w299] mode=indexing
          tunnel: w284 -> [w298] mode=indexing
          tunnel: w283 -> [w297] mode=indexing
          tunnel: w281 -> [w293]
          tunnel: w280 -> [w292]
          tunnel: w279 -> [w291]
          tunnel: "Color Table" -> [w290]
          n131 = call "EncodeInLine.vi"("Look Up Table"=w291, "Final Sector Image Size"=w301, "Range Params"=w302, "Header In"=w300, 5:w299, "PSA Value"=w293, "intercept"=w298, "thresholds"=w292, "midband fit"=w297) -> ("Scale Score"=w294:dbl[][], "Colored MB"=w296:dbl[][], "colored Int"=w295:dbl[][], "Colored Score"=w289:dbl[][])  [unwired: 1 in, 6 out]
          n132 = call "SaveScoreImages.vi"("Color Table"=w290, "Save Directory"=w304, "FileName"=w303, "Colored Score"=w289, "colored Int"=w295, "Colored MB"=w296, "Scaled Score"=w294) -> ()  [unwired: 5 out]
        }
      }
      event "Rescale Thresh": Value Change {
        n133 = event-data() -> ()  [unwired: 1 in, 5 out]
        n134 = local read "max value"() -> (w308:dbl)
        n135 = local read "min value"() -> (w307:dbl)
        n136 = Round Toward +Infinity(x=w308) -> (ceil(x): smallest int >= x=w306:dbl)
        n137 = Round Toward -Infinity(1:w307) -> (0:w305:dbl)
        n138 = property on="T1" class="Slide (strict)"("Scale.Maximum"=w306, "Scale.Minimum"=w305) -> ()  [unwired: 2 in, 2 out]
        n139 = property on="T2" class="Slide (strict)"("Scale.Maximum"=w306, "Scale.Minimum"=w305) -> ()  [unwired: 2 in, 2 out]
        n140 = property on="T3" class="Slide (strict)"("Scale.Maximum"=w306, "Scale.Minimum"=w305) -> ()  [unwired: 2 in, 2 out]
        n141 = property on="T4" class="Slide (strict)"("Scale.Maximum"=w306, "Scale.Minimum"=w305) -> ()  [unwired: 2 in, 2 out]
        n142 = property on="T5" class="Slide (strict)"("Scale.Maximum"=w306, "Scale.Minimum"=w305) -> ()  [unwired: 2 in, 2 out]
      }
      event "ExitSendCmd": Value Change {
        n143 = event-data() -> ()  [unwired: 1 in, 5 out]
      }
    }
  }
